vi "insertBeforeExtension.vi"(8 "error in (no error)":errorcluster, 9 "Insert":string, 10 "Filepath":path) -> (0 "error out":errorcluster, 2 "Filepath with insert":path)   [LabVIEW 2017]
doc: "Insert text right before file extension in path, and return modified path"
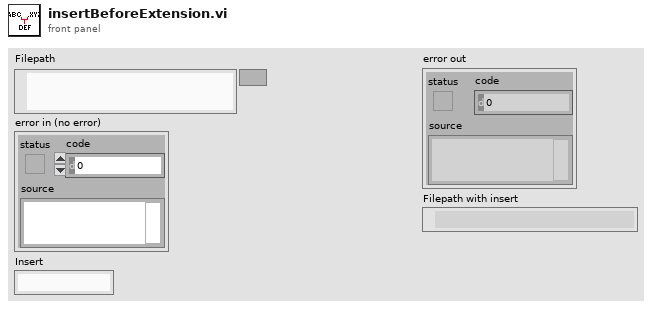
[diagram p1: front panel]
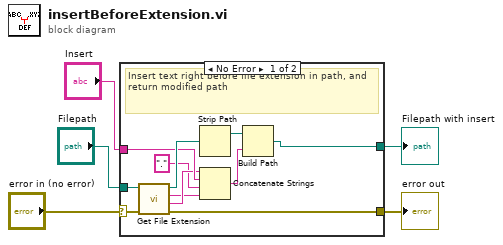
[diagram p0: block diagram]
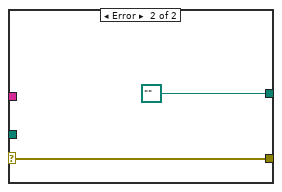
[diagram p2: hidden frame]
diagram:
  n1 = case shown="No Error" "error in (no error)" {
    selector: "error in (no error)" -> [w6 w18]
    tunnel: "Filepath" -> [w16 _]
    tunnel: [w15 w18] -> w4
    tunnel: "Insert" -> [w13 _]
    tunnel: [w7 path "" ("appended path")] -> w2
    frame No Error {
      # "Insert text right before file extension in path, and return modified path"
      n2 = call <vilib>:"Get File Extension.vi"("error in (no error)"=w6, "file"=w16) -> ("error out"=w15:errorcluster, "filename without extension"=w12:string, "lowercase file extension"=w10:string, "dup file"=w14:path)  [unwired: 5 in, 1 out]
      n3 = Strip Path(path=w14) -> (stripped path=w8:path)  [unwired: 1 out]
      n4 = Concatenate Strings(w12, w13, "." ("string"), w10) -> (w9:string)
      n5 = Build Path(base path=w8, name or relative path=w9) -> (appended path=w7:path)
    }
    frame Error {
    }
  }
  "error out" <- w4
  "Filepath with insert" <- w2
